vi "16bitScalebar.vi"(2 "Boolean":bool) -> (0 "Image Out":T1)   [LabVIEW 2009]
uses:
  <vilib>/vision/Image Controls.llb/IMAQ Image.ctl
panel:
  in  "Image Type":u32(ring)=1 items=["8 bits", "16 bits", "Float", "Complex", "RGB", "HSL"]
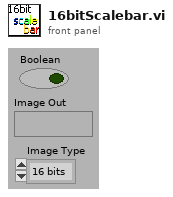
[diagram p1: front panel]
types:
  T1 = typedef "IMAQ Image.ctl" = refnum<image>
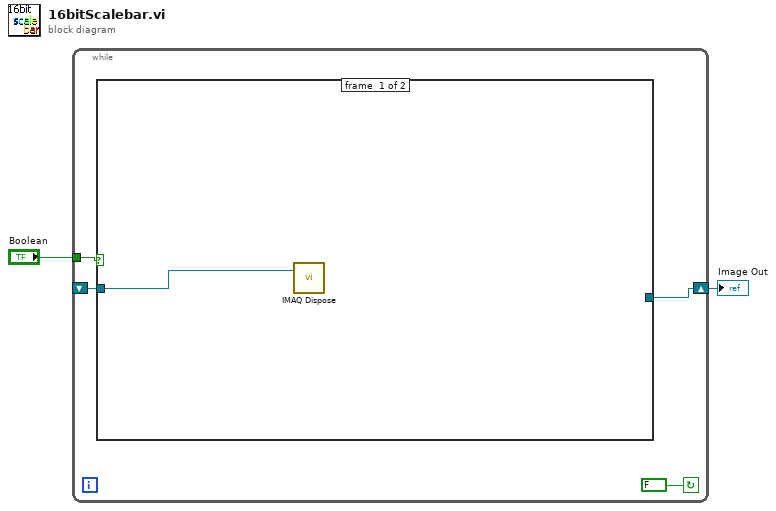
[diagram p0: block diagram]
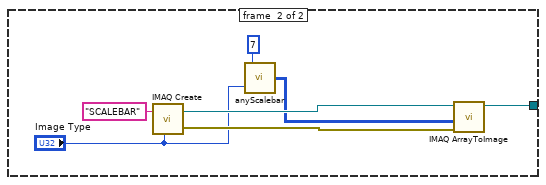
[diagram p2: hidden frame]
diagram:
  n1 = while {
    shift-right: [w6] -> w1
    shift-left: _ -> [w5]
    tunnel: "Boolean" -> [w3]
    stop <- FALSE continue-if-true
    n2 = case shown="True" w3 {
      tunnel: [_ w9] -> w6
      tunnel: w5 -> [w7 _]
      frame #0 {
        n3 = call "IMAQ Dispose"("Image"=w7) -> ()  [unwired: 5 in, 1 out]
      }
      frame #1 {
        n4 = call "IMAQ Create"("Image Name"="SCALEBAR", "Image Type"="Image Type") -> ("New Image"=w11:T1, "error out"=w12:errorcluster)  [unwired: 3 in]
        n5 = call "anyScalebar.vi"("Image Type"="Image Type", "Window Number"=7) -> ("Image Pixels (I16)"=w10:i16[][])
        n6 = call "IMAQ ArrayToImage"("error in (no error)"=w12, "Image Pixels (I16)"=w10, "Image"=w11) -> ("Image Out"=w9:T1)  [unwired: 7 in, 1 out]
      }
    }
  }
  "Image Out" <- w1
